vi "FTW-Logger-AddRecord.vi"(0 "FTW Logger Connector":refnum<class "FTW-Logger.lvclass">, 5 "Event Type":string, 7 "Event Data":string, 9 "Source (unwired for call chain)":string="CallChain", 11 "error in":errorcluster) -> (4 "FTW Logger Connector out":refnum<class "FTW-Logger.lvclass">, 6 "Serialized Event":string, 15 "error out":errorcluster)   [LabVIEW 2013, in "FTW-Logger.lvclass"]
doc: "This method queues an event to be logged by the Logger associated with the LoggerID."
uses:
  FTW-Logger.lvclass
  connector/FTW-Actor-Connector.lvclass
panel:
  # "Inputs"
  # "Outputs"
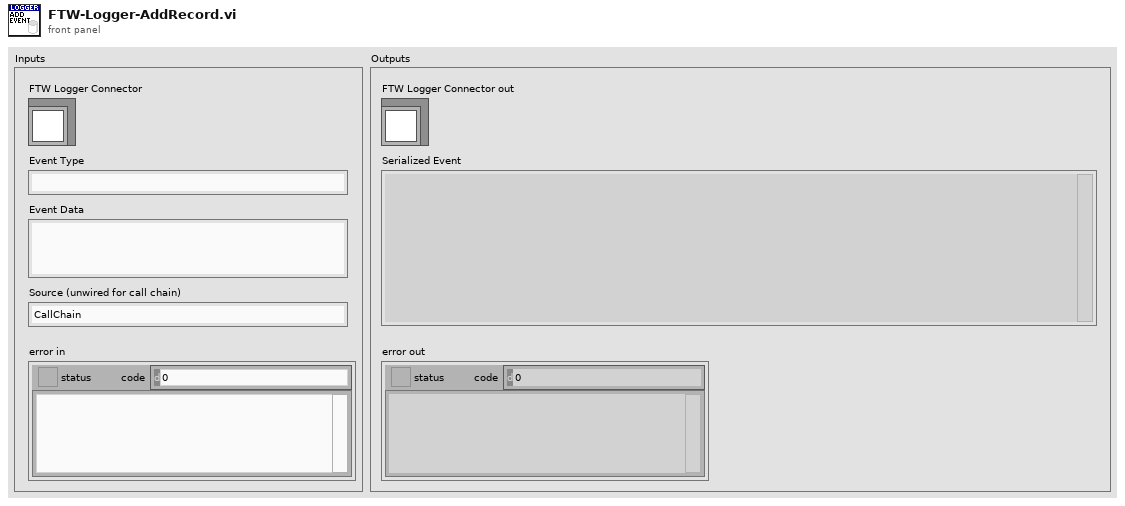
[diagram p1: front panel]
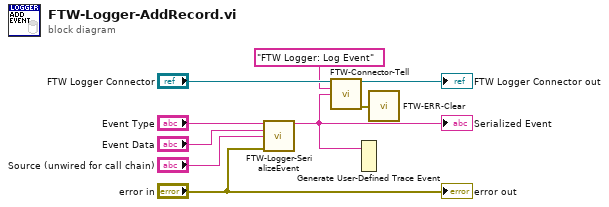
[diagram p0: block diagram]
diagram:
  n1 = call "FTW-Logger-SerializeEvent.vi"("Event Type"="Event Type", "Event Data"="Event Data", "Source (unwired for call chain, Empty to omit)"="Source (unwired for call chain)", "Error to Log"="error in") -> ("Serialized Event"=w3:string)  [unwired: 11 in]
  "Serialized Event" <- w3
  n2 = call "FTW-Connector-Tell.vi"("FTW Actor Connector"="FTW Logger Connector", "Message Header"="FTW Logger: Log Event" ("Parameter"), "Message Body"=w3) -> ("FTW Actor Connector out"=→"FTW Logger Connector out":refnum<class "FTW-Logger.lvclass">, "error out"=w2:errorcluster)  [unwired: 10 in, 1 out]
  n3 = Generate User-Defined Trace Event(2:w3) -> ()  [unwired: 1 in]
  n4 = call "FTW-ERR-Clear.vi"("error to snuff"=w2) -> ()  [unwired: 1 out]
  "error out" <- "error in"
